vi "DAQ Relay States - Retrieve.vi"(0 "TSM Context":T3, 11 "error in (no error)":errorcluster) -> (4 "DAQ States - Out":T1[](array[typedef]) {"Relay Action" items=["Open Relay"=20, "Close Relay"=21]}, 6 "DAQ Relay Names String":string[](array[string]), 15 "error out":errorcluster)   [LabVIEW 2019]
uses:
  <vilib>/NI_TestStand_SemiconductorModule/NI_TestStand_Semiconductor_Module.lvlibp/PinMap/General/SemiconductorModuleContext.ctl
  typedefs/DAQ Relay Pins.ctl
  <vilib>/NI_TestStand_SemiconductorModule/NI_TestStand_Semiconductor_Module.lvlibp/1abvi3w/instr.lib/niSwitch/niswitch.llb/niSwitch Relay Action.ctl
  TSM Context Data Access/Public/Properties/DAQ Relay States - Read.vi
  TSM Context Data Access/TSM Context Data Access.lvclass
  <vilib>/NI_TestStand_SemiconductorModule/NI_TestStand_Semiconductor_Module.lvlibp
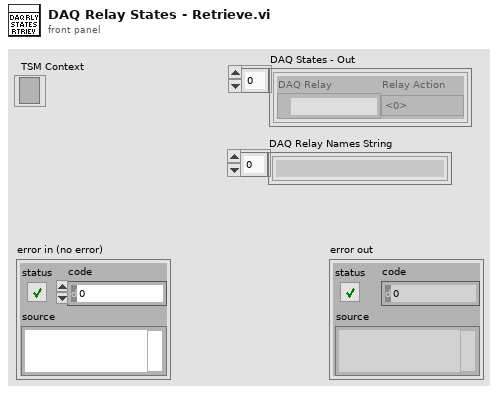
[diagram p1: front panel]
types:
  T1 = typedef "DAQ Relay Pins.ctl" = cluster{"DAQ Relay":tag, "Relay Action":T2}
  T2 = typedef "NI_TestStand_Semiconductor_Module.lvlibp/niSwitch Relay Action.ctl" = i32
  T3 = typedef "NI_TestStand_Semiconductor_Module.lvlibp/SemiconductorModuleContext.ctl" = refnum<k7>
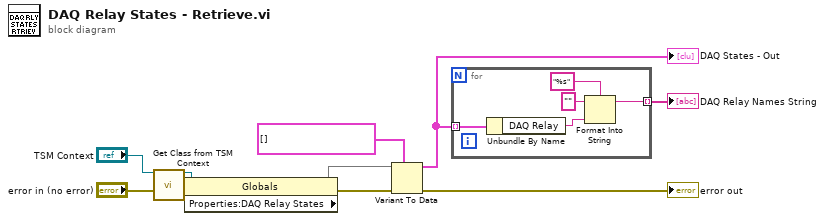
[diagram p0: block diagram]
diagram:
  n1 = call "Get Class from TSM Context.vi"("TSM Context"="TSM Context") -> ("Global Memory Class"=w8:refnum<class "TSM Context Data Access.lvclass">)  [unwired: 14 in]
  n2 = property class="Globals"(reference=w8, error in="error in (no error)") -> (error out=w7:errorcluster, "Properties:DAQ Relay States"=w5)  [unwired: 1 out]
  n3 = Variant To Data(error in=w7, type=T1[] [], Variant=w5) -> (data=w1:T1[], error out=→"error out":errorcluster)
  "DAQ States - Out" <- w1
  n4 = for {
    tunnel: w1 -> [w14] mode=indexing
    tunnel: [w10] -> w2 mode=indexing
    n5 = Unbundle By Name(w14) -> ("DAQ Relay"=w11:tag)
    n6 = Format Into String(format string="%s", initial string="", w11) -> (resulting string=w10:string)  [unwired: 1 in, 1 out]
  }
  "DAQ Relay Names String" <- w2
